vi "Blit Surface.vi"(6 "Destination Rectangle Pointer":u32 format="%.0x", 8 "error in":errorcluster, 9 "Destination Surface Pointer":u32 format="%.0x", 10 "Source Rectangle Pointer":u32 format="%.0x", 11 "Source Surface Pointer":u32 format="%.0x") -> (0 "error out":errorcluster, 3 "Return":i32)   [LabVIEW 2014, in "LibSDL2.lvlib"]
uses:
  LibSDL2.lvlib
  DLL/SDL2.dll
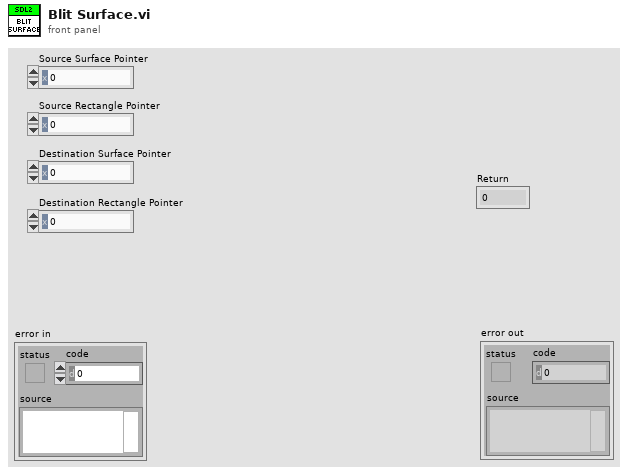
[diagram p1: front panel]
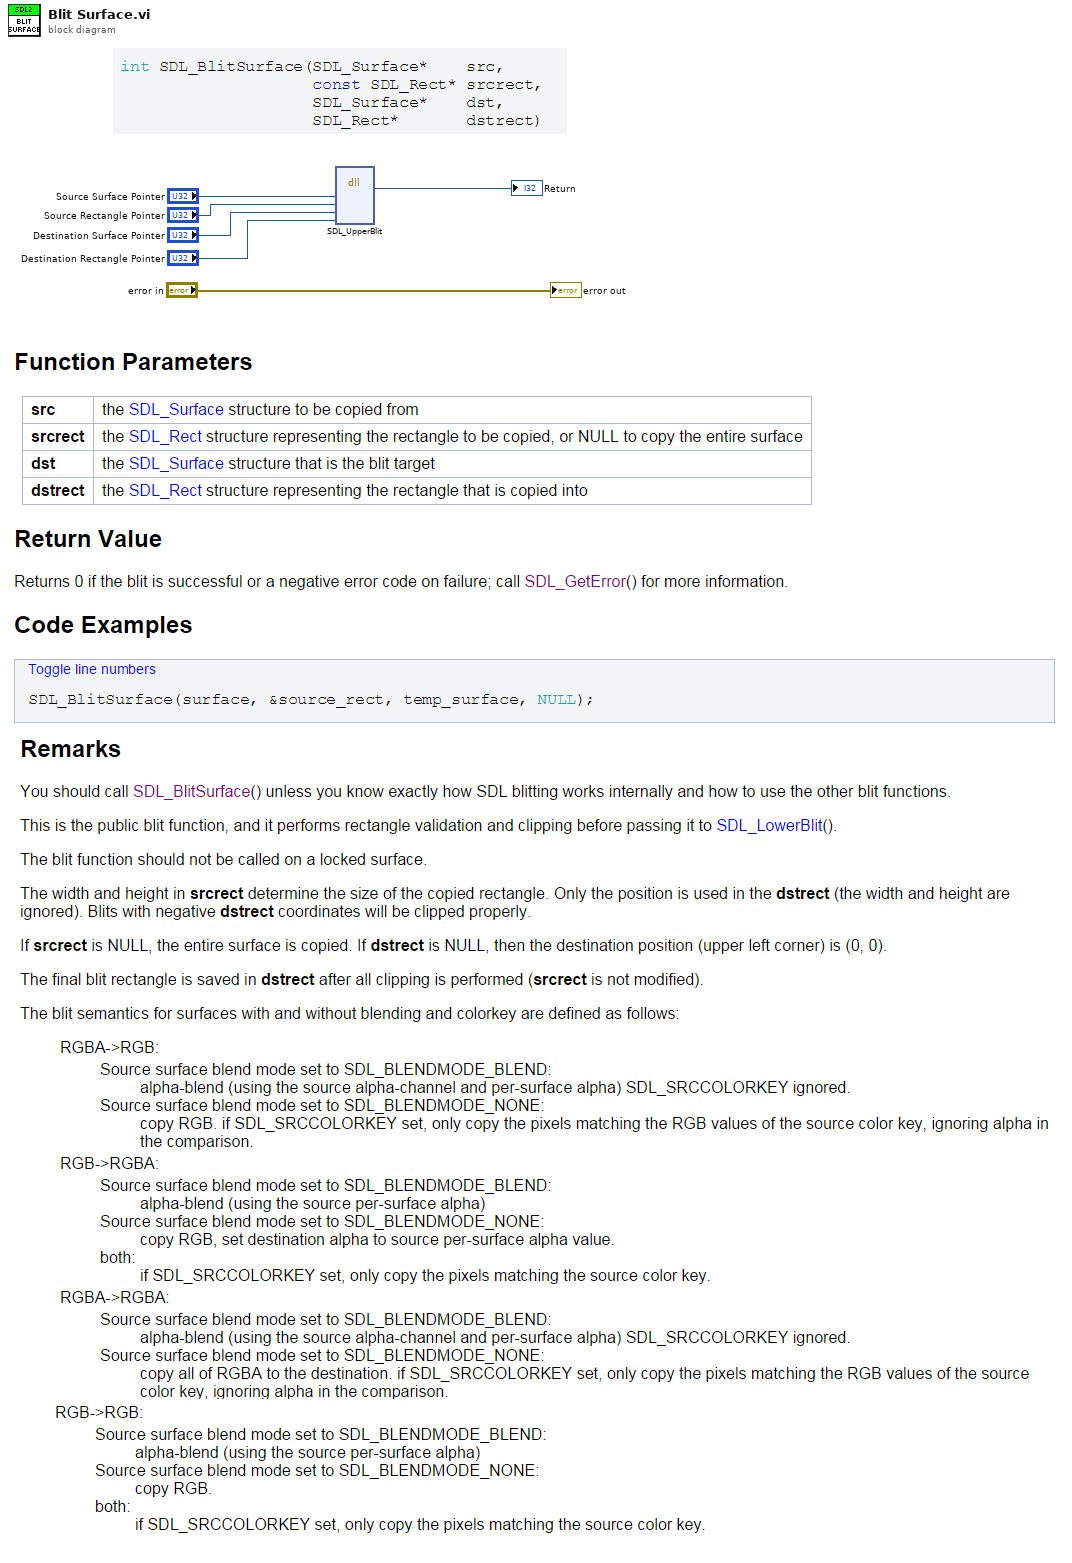
[diagram p0: block diagram]
diagram:
  n1 = dll-call lib="C:/dev/PGS/LabSDL2/Source/LibSDL2 Wrapper/DLL/SDL2.dll" fn="SDL_UpperBlit"("src"="Source Surface Pointer", "srcrect"="Source Rectangle Pointer", "dst"="Destination Surface Pointer", "dstrect"="Destination Rectangle Pointer") -> ("return type"=→"Return":i32)  [unwired: 7 in, 2 out]
  "error out" <- "error in"
